vi "adcTOrev.vi"(11 "ADC count":dbl) -> (3 "Estimated Possition":dbl)   [LabVIEW 2019]
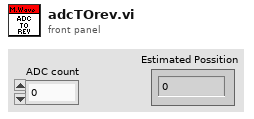
[diagram p1: front panel]
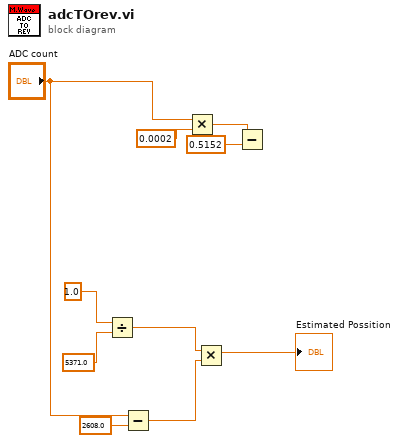
[diagram p0: block diagram]
diagram:
  n1 = Divide(x=1.0, y=5371.0) -> (x/y=w5:dbl)
  n2 = Subtract(x="ADC count", y=2608.0) -> (x-y=w4:dbl)
  n3 = Multiply(x="ADC count", y=0.0002) -> (x*y=w9:dbl)
  n4 = Multiply(x=w5, y=w4) -> (x*y=→"Estimated Possition":dbl)
  n5 = Subtract(x=w9, y=0.5152) -> ()  [unwired: 1 out]
